vi "Get Image Date.vi"(8 "error in (no error)":errorcluster, 11 "Header in":refnum<class "Header.lvclass">) -> (0 "error out":errorcluster, 3 "Header out":refnum<class "Header.lvclass">)   [LabVIEW 2018, in "Header.lvclass"]
uses:
  Header.lvclass
  C:/Users/observer/Desktop/SPARC4_ACS/SPARC4_ACS/Simulated_Header/Simulated_Header.lvclass
  Simulated_Header/Simulated_Header.lvclass
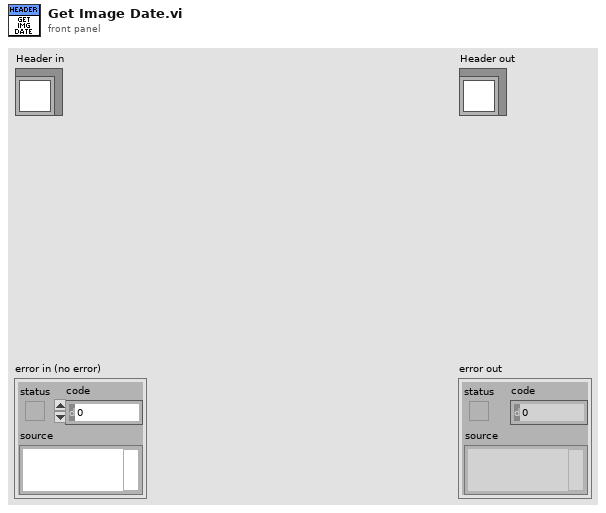
[diagram p1: front panel]
types:
  T1 = typedef "SYSTEMTIME structure typedef.ctl" = cluster{"Year":u16, "Month":u16, "DayOfWeek":u16, "Date":u16, "Hour":u16, "Minute":u16, "Second":u16, "Milliseconds":u16}
  T2 = cluster{"FILENAME":cluster{"Name":string, "Value":string, "Comment":string}, "OBSERVER":cluster{"Name":string, "Value":string, "Comment":string}, "PROGRID":cluster{"Name":string, "Value":string, "Comment":string}, "OBJECT":cluster{"Name":string, "Value":string, "Comment":string}, "NIGHTDIR":cluster{"Name":string, "Value":string, "Comment":string}, "CHANNEL":cluster{"Name":string, "Value":string, "Comment":string}, "INSTRUME":cluster{"Name":string, "Value":string, "Comment":string}, "NEXPSEQ":cluster{"Name":string, "Value":u16, "Comment":string}, "SEQINDEX":cluster{"Name":string, "Value":u16, "Comment":string}, "OBSTYPE":cluster{"Name":string, "Value":string, "Comment":string}, "READMOD":cluster{"Name":string, "Value":string, "Comment":string}, "READMODE":cluster{"Name":string, "Value":string, "Comment":string}, "ACQMODE":cluster{"Name":string, "Value":string, "Comment":string}, "PREAMP":cluster{"Name":string, "Value":string, "Comment":string}, "READOUT":cluster{"Name":string, "Value":string, "Comment":string}, "VSHIFT":cluster{"Name":string, "Value":string, "Comment":string}, "TRIGGER":cluster{"Name":string, "Value":string, "Comment":string}, "EMMODE":cluster{"Name":string, "Value":string, "Comment":string}, "EMGAIN":cluster{"Name":string, "Value":u16, "Comment":string}, "VBIN":cluster{"Name":string, "Value":u16, "Comment":string}, "HBIN":cluster{"Name":string, "Value":u16, "Comment":string}, "INITLIN":cluster{"Name":string, "Value":u16, "Comment":string}, "INITCOL":cluster{"Name":string, "Value":u16, "Comment":string}, "FINALLIN":cluster{"Name":string, "Value":u16, "Comment":string}, "FINALCOL":cluster{"Name":string, "Value":u16, "Comment":string}, "KSERLEN":cluster{"Name":string, "Value":u16, "Comment":string}, "SHUTTER":cluster{"Name":string, "Value":string, "Comment":string}, "OPENSHT":cluster{"Name":string, "Value":u16, "Comment":string}, "CLOSESHT":cluster{"Name":string, "Value":u16, "Comment":string}, "DATE":cluster{"Name":string, "Value":string, "Comment":string}, "GAIN":cluster{"Name":string, "Value":dbl, "Comment":string}, "GAINERR":cluster{"Name":string, "Value":dbl, "Comment":string}, "RDNOISE":cluster{"Name":string, "Value":dbl, "Comment":string}, "RNOISERR":cluster{"Name":string, "Value":dbl, "Comment":string}, "SKYFIBER":cluster{"Name":string, "Value":string, "Comment":string}, "CALFIBER":cluster{"Name":string, "Value":string, "Comment":string}, "UTDATE":cluster{"Name":string, "Value":string, "Comment":string}, "LOCTIME":cluster{"Name":string, "Value":string, "Comment":string}, "MJD":cluster{"Name":string, "Value":dbl, "Comment":string}, "OBSLON":cluster{"Name":string, "Value":string, "Comment":string}, "OBSLAT":cluster{"Name":string, "Value":string, "Comment":string}, "OBSALT":cluster{"Name":string, "Value":dbl, "Comment":string}, "EXPTIME":cluster{"Name":string, "Value":dbl, "Comment":string}, "TELRA":cluster{"Name":string, "Value":string, "Comment":string}, "TELDEC":cluster{"Name":string, "Value":string, "Comment":string}, "RA":cluster{"Name":string, "Value":string, "Comment":string}, "DEC":cluster{"Name":string, "Value":string, "Comment":string}, "RA_DEG":cluster{"Name":string, "Value":dbl, "Comment":string}, "DEC_DEG":cluster{"Name":string, "Value":dbl, "Comment":string}, "EPOCH":cluster{"Name":string, "Value":dbl, "Comment":string}, "HA":cluster{"Name":string, "Value":string, "Comment":string}, "HAD":cluster{"Name":string, "Value":dbl, "Comment":string}, "AIRMASS":cluster{"Name":string, "Value":dbl, "Comment":string}, "AMSTART":cluster{"Name":string, "Value":dbl, "Comment":string}, "AMEND":cluster{"Name":string, "Value":dbl, "Comment":string}, "XOFFSET":cluster{"Name":string, "Value":dbl, "Comment":string}, "YOFFSET":cluster{"Name":string, "Value":dbl, "Comment":string}, "PA":cluster{"Name":string, "Value":dbl, "Comment":string}, "CAMFOC":cluster{"Name":string, "Value":string, "Comment":string}, "TELFOC":cluster{"Name":string, "Value":dbl, "Comment":string}, "TCSUT":cluster{"Name":string, "Value":string, "Comment":string}, "TCSST":cluster{"Name":string, "Value":string, "Comment":string}, "MOONDIST":cluster{"Name":string, "Value":dbl, "Comment":string}, "MOONALT":cluster{"Name":string, "Value":dbl, "Comment":string}, "MOONPHAS":cluster{"Name":string, "Value":string, "Comment":string}, "ADC":cluster{"Name":string, "Value":string, "Comment":string}, "ADCSPEED":cluster{"Name":string, "Value":dbl, "Comment":string}, "CALMIRR":cluster{"Name":string, "Value":string, "Comment":string}, "GUIDING":cluster{"Name":string, "Value":string, "Comment":string}, "GUIDTEXP":cluster{"Name":string, "Value":dbl, "Comment":string}, "GUIDFREQ":cluster{"Name":string, "Value":dbl, "Comment":string}, "GUIDOBJX":cluster{"Name":string, "Value":dbl, "Comment":string}, "GUIDOBJY":cluster{"Name":string, "Value":dbl, "Comment":string}, "AVGYCORR":cluster{"Name":string, "Value":dbl, "Comment":string}, "AVGXCORR":cluster{"Name":string, "Value":dbl, "Comment":string}, "GFOCUS":cluster{"Name":string, "Value":dbl, "Comment":string}, "THARLAMP":cluster{"Name":string, "Value":string, "Comment":string}, "HALLAMP":cluster{"Name":string, "Value":string, "Comment":string}, "AGITATOR":cluster{"Name":string, "Value":string, "Comment":string}, "THARMIRR":cluster{"Name":string, "Value":string, "Comment":string}, "DSTATUS":cluster{"Name":string, "Value":string, "Comment":string}, "DPOS":cluster{"Name":string, "Value":dbl, "Comment":string}, "DTEMP":cluster{"Name":string, "Value":dbl, "Comment":string}, "DHUM":cluster{"Name":string, "Value":string, "Comment":string}, "DLAMP":cluster{"Name":string, "Value":string, "Comment":string}, "DFLAT":cluster{"Name":string, "Value":string, "Comment":string}, "TEMPEXT":cluster{"Name":string, "Value":string, "Comment":string}, "PRESSURE":cluster{"Name":string, "Value":string, "Comment":string}, "HUMIDITY":cluster{"Name":string, "Value":string, "Comment":string}, "WINDDIR":cluster{"Name":string, "Value":string, "Comment":string}, "WINSPEED":cluster{"Name":string, "Value":dbl, "Comment":string}, "SHTTTL":cluster{"Name":string, "Value":string, "Comment":string}, "COOLER":cluster{"Name":string, "Value":string, "Comment":string}, "TEMP":cluster{"Name":string, "Value":u16, "Comment":string}, "TEMPST":cluster{"Name":string, "Value":string, "Comment":string}, "SERN":cluster{"Name":string, "Value":u16, "Comment":string}, "COMMENT":cluster{"Name":string, "Value":string, "Comment":string}, "SIMPLE":cluster{"Name":string, "Value":string, "Comment":string}, "BITPIX":cluster{"Name":string, "Value":u16, "Comment":string}, "EXTEND":cluster{"Name":string, "Value":string, "Comment":string}, "FRAME_T":cluster{"Name":string, "Value":string, "Comment":string}, "VCLOCK":cluster{"Name":string, "Value":string, "Comment":string}, "ADCHNNL":cluster{"Name":string, "Value":u16, "Comment":string}, "JD":cluster{"Name":string, "Value":dbl, "Comment":string}, "SD":cluster{"Name":string, "Value":string, "Comment":string}, "FILTER":cluster{"Name":string, "Value":string, "Comment":string}, "ACSVRSN":cluster{"Name":string, "Value":string, "Comment":string}, "CTRLINTER":cluster{"Name":string, "Value":string, "Comment":string}, "NAXIS3":cluster{"Name":string, "Value":u32, "Comment":string}, "NAXIS2":cluster{"Name":string, "Value":u32, "Comment":string}, "NAXIS1":cluster{"Name":string, "Value":u32, "Comment":string}, "NAXIS":cluster{"Name":string, "Value":u32, "Comment":string}}
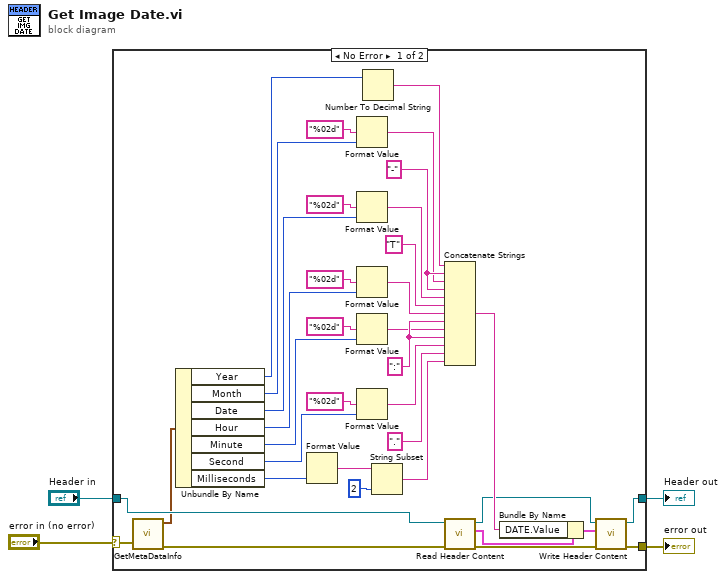
[diagram p0: block diagram]
diagram:
  n1 = case shown="No Error" "error in (no error)" {
    selector: "error in (no error)" -> [w6 w42]
    tunnel: [w12 w42] -> w2
    tunnel: [w11 w41] -> w1
    tunnel: "Header in" -> [w16 w41]
    frame No Error {
      w38 = ":"
      w39 = "-"
      n2 = call <userlib>:"GetMetaDataInfo.vi"("error in (no error)"=w6) -> ("SYSTEMTIME"=w7:T1, "error out"=w5:errorcluster)  [unwired: 1 in, 2 out]
      n3 = Unbundle By Name(w7) -> ("Year"=w40:u16, "Month"=w31:u16, "Date"=w30:u16, "Hour"=w29:u16, "Minute"=w28:u16, "Second"=w27:u16, "Milliseconds"=w8:u16)
      n4 = Format Value(value (0)=w8) -> (output string=w26:string)  [unwired: 2 in]
      n5 = Format Value(format string="%02d", value (0)=w31) -> (output string=w24:string)  [unwired: 1 in]
      n6 = Format Value(format string="%02d", value (0)=w30) -> (output string=w23:string)  [unwired: 1 in]
      n7 = Format Value(format string="%02d", value (0)=w29) -> (output string=w21:string)  [unwired: 1 in]
      n8 = Format Value(format string="%02d", value (0)=w28) -> (output string=w20:string)  [unwired: 1 in]
      n9 = Format Value(format string="%02d", value (0)=w27) -> (output string=w19:string)  [unwired: 1 in]
      n10 = Number To Decimal String(number=w40) -> (decimal integer string=w25:string)  [unwired: 1 in]
      n11 = String Subset(string=w26, length (rest)=2 ("offset (0)")) -> (substring=w9:string)  [unwired: 1 in]
      n12 = Concatenate Strings(w25, w39, w24, w39, w23, "T", w21, w38, w20, w38, w19, ".", w9) -> (w18:string)
      n13 = call "Read Header Content.vi"("error in (no error)"=w5, "Simulated_Header in"=w16) -> ("error out"=w13:errorcluster, "Header Content"=w17:T2, "Simulated_Header out"=w15:refnum<class "Header.lvclass">)  [unwired: 7 in]
      n14 = Bundle By Name(cluster=w17, "DATE.Value"=w18) -> (w14:T2)
      n15 = call "Write Header Content.vi"("error in (no error)"=w13, "Header Content"=w14, "Simulated_Header in"=w15) -> ("error out"=w12:errorcluster, "Simulated_Header out"=w11:refnum<class "Header.lvclass">)  [unwired: 7 in]
    }
    frame Error {
    }
  }
  "error out" <- w2
  "Header out" <- w1
